vi "CAN Send and Receive.vi"(5 "CAN Timeout (ms)":i32=20, 6 "Receive Message ID Mask":u32=268435455 format="%x", 7 "CAN Max Retries":i32=5, 8 "error in (no error)":errorcluster, 9 "Send Data":u8[](array[numeric]), 10 "Receive Message ID":u32, 11 "Send Message ID":u32) -> (0 "error out":errorcluster, 3 "Receive Data":u8[](array[numeric]))   [LabVIEW 2023]
uses:
  0a2af276-7e4e-4a0d-beba-9fb8726c08b7.vi
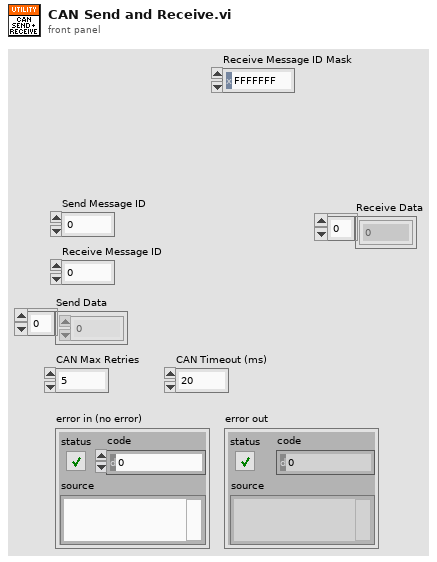
[diagram p1: front panel]
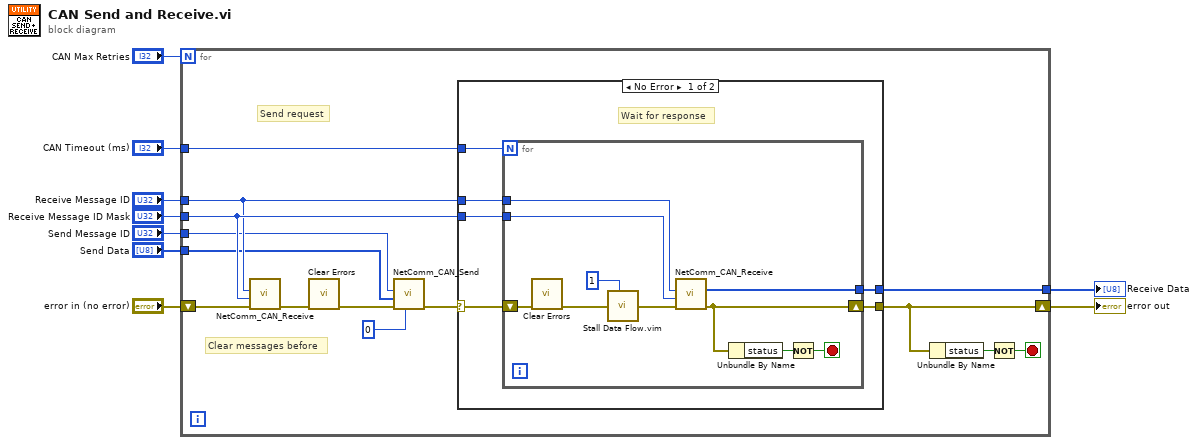
[diagram p0: block diagram]
diagram:
  n1 = for {
    N: "CAN Max Retries" -> [_]
    tunnel: [w22] -> w8
    shift-right: [w21] -> w6
    shift-left: "error in (no error)" -> [w16]
    tunnel: "Receive Message ID Mask" -> [w14]
    tunnel: "Receive Message ID" -> [w13]
    tunnel: "CAN Timeout (ms)" -> [w12]
    tunnel: "Send Data" -> [w11]
    tunnel: "Send Message ID" -> [w10]
    stop <- w18 stop-if-true
    # "Clear messages before"
    # "Send request"
    n2 = call <vilib>:"NetComm_CAN_Receive.vi"("error in (no error)"=w16, "Message ID Mask"=w14, "Message ID"=w13) -> ("error out"=w15:errorcluster)  [unwired: 8 out]
    n3 = call <vilib>:"Clear Errors.vi"("error in (no error)"=w15) -> ("error out"=w17:errorcluster)  [unwired: 5 in, 1 out]
    n4 = call <vilib>:"NetComm_CAN_Send.vi"("Period (ms)"=0, "error in (no error)"=w17, "Data"=w11, "Message ID"=w10) -> ("error out"=w19:errorcluster)  [unwired: 7 out]
    n5 = case shown="No Error" w19 {
      selector: w19 -> [w27 w40]
      tunnel: [w29 _] -> w22
      tunnel: [w28 w40] -> w21
      tunnel: w14 -> [w26 _]
      tunnel: w13 -> [w25 _]
      tunnel: w12 -> [w24 _]
      frame No Error {
        # "Wait for response"
        n6 = for {
          N: w24 -> [_]
          tunnel: [w39] -> w29
          shift-right: [w35] -> w28
          shift-left: w27 -> [w38]
          tunnel: w26 -> [w31]
          tunnel: w25 -> [w30]
          stop <- w33 stop-if-true
          n7 = call <vilib>:"Clear Errors.vi"("error in (no error)"=w38) -> ("error out"=w32:errorcluster)  [unwired: 5 in, 1 out]
          n8 = call "Stall Data Flow.vim"("value in"=w32, "milliseconds to wait"=u32 1) -> ("value out"=w37:errorcluster)  [unwired: 1 out]
          n9 = call <vilib>:"NetComm_CAN_Receive.vi"("error in (no error)"=w37, "Message ID Mask"=w31, "Message ID"=w30) -> ("error out"=w35:errorcluster, "Data"=w39:u8[])  [unwired: 7 out]
          n10 = Unbundle By Name(w35) -> ("status"=w34:bool)
          n11 = Not(x=w34) -> (.not. x?=w33:bool)
        }
      }
      frame Error {
      }
    }
    n12 = Unbundle By Name(w21) -> ("status"=w20:bool)
    n13 = Not(x=w20) -> (.not. x?=w18:bool)
  }
  "Receive Data" <- w8
  "error out" <- w6
